vi "configure channel.vi"(7 "user event":T1, 8 "error in":errorcluster, 9 "line":T2, 10 "engine configuration in":refnum<class "engine configuration.lvclass">, 11 "Scan Engine configuration in":refnum<class "Scan Engine configuration.lvclass">) -> (0 "error out":errorcluster, 2 "engine configuration out":refnum<class "engine configuration.lvclass">, 3 "Scan Engine configuration out":refnum<class "Scan Engine configuration.lvclass">)   [LabVIEW 2013, in "Scan Engine editor node.lvclass"]
uses:
  Scan Engine editor node.lvclass
  module/configuration/Scan Engine configuration.lvclass
  <vilib>/NI/Module Execution Interface/Engine Configuration/engine configuration.lvclass
  table line.ctl
  <vilib>/NI/Tag Bus Module Framework/channel/TBM channel.lvclass
  <vilib>/NI/Configuration Framework/Node/UserEventRef.ctl
  <vilib>/NI/Configuration Framework/Controls/EventCluster.ctl
  <vilib>/NI/Configuration Framework/serializable configuration/NISE_CEF_serializable configuration.lvclass/NISE_CEF_serializable configuration.ctl
  <vilib>/NI/Tag Bus/tag/tag descriptor.lvclass/tag descriptor.ctl
  <vilib>/Utility/LVClass/Get LV Class Name.vi
  <vilib>/NI/Configuration Framework/error generator/NISE_error generator.vi
  <vilib>/NI/Tag Bus/tag/tag descriptor.lvclass
  <vilib>/NI/Configuration Framework/NISE_CEF_TreeControl.lvlib
  <vilib>/NI/Configuration Framework/serializable configuration/NISE_CEF_serializable configuration.lvclass
  <vilib>/NI/Configuration Framework/Node/NISE_CEF_Node.lvclass
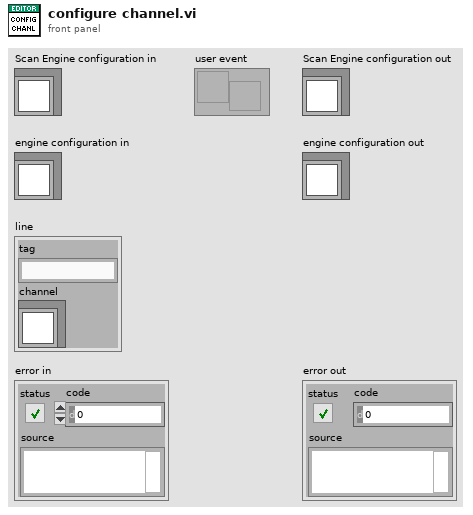
[diagram p1: front panel]
types:
  T1 = typedef "NISE_CEF_Node.lvclass/UserEventRef.ctl" = refnum<user-event>
  T2 = typedef "Scan Engine editor node.lvclass/table line.ctl" = cluster{"tag":string, "channel":refnum<class "TBM channel.lvclass">}
  T3 = typedef "NISE_CEF_TreeControl.lvlib/EventCluster.ctl" = cluster{"command":string, "data":string}
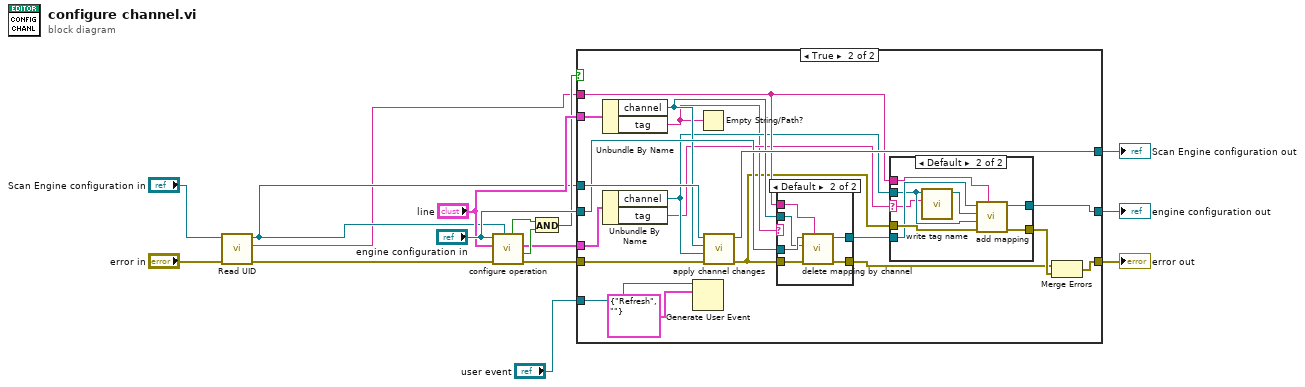
[diagram p0: block diagram]
diagram:
  n1 = call <vilib>:"Read UID.vi"("error in"="error in", "configuration in"="Scan Engine configuration in") -> ("error out"=w4:errorcluster, "instance id"=w1:string, "configuration out"=w2:refnum<class "Scan Engine configuration.lvclass">)  [unwired: 7 in]
  n2 = call "configure operation.vi"("Scan Engine configuration"=w2, "error in"=w4, "line item in"="line", "engine configuration in"="engine configuration in") -> ("error out"=w7:errorcluster, "success"=w12:bool, "line item out"=w8:T2, "changed"=w11:bool)  [unwired: 4 in]
  n3 = And(x=w11, y=w12) -> (x .and. y?=w13:bool)
  n4 = case shown="True" w13 {
    tunnel: [w18 w24] -> w10
    tunnel: [w19 w28] -> w15
    tunnel: "engine configuration in" -> [w19 w33]
    tunnel: w7 -> [w18 w35]
    tunnel: w8 -> [_ w38]
    tunnel: w2 -> [w17 w37]
    tunnel: [w17 w34] -> w9
    tunnel: w1 -> [_ w30]
    tunnel: "line" -> [_ w36]
    tunnel: "user event" -> [_ w20]
    frame False {
    }
    frame True {
      n5 = Unbundle By Name(w36) -> ("channel"=w32:refnum<class "TBM channel.lvclass">, "tag"=w25:string)
      n6 = Unbundle By Name(w38) -> ("channel"=w27:refnum<class "TBM channel.lvclass">, "tag"=w26:string)
      n7 = Generate User Event(user event=w20, event data cluster=T3 {"command"="Refresh", "data"=""} ("event data")) -> ()  [unwired: 2 in, 2 out]
      n8 = Empty String/Path?(string/path=w25) -> ()  [unwired: 1 out]
      n9 = call "apply channel changes.vi"("error in"=w35, "new"=w27, "old"=w32, "Scan Engine configuration"=w37) -> ("error out"=w22:errorcluster, "Scan Engine configuration out"=w34:refnum<class "Scan Engine configuration.lvclass">)  [unwired: 6 in]
      n10 = case shown="Default" w25 {
        tunnel: w22 -> [w39 w46]
        tunnel: w33 -> [w40 w45]
        tunnel: w32 -> [_ w44]
        tunnel: [w39 w43] -> w23
        tunnel: w30 -> [_ w42]
        tunnel: [w40 w41] -> w29
        frame "" {
        }
        frame Default {
          n11 = call <vilib>:"delete mapping by channel.vi"("owner ID"=w42, "error in"=w46, "channel"=w44, "engine configuration in"=w45) -> ("error out"=w43:errorcluster, "engine configuration out"=w41:refnum<class "engine configuration.lvclass">)  [unwired: 6 in]
        }
      }
      n12 = case shown="Default" w26 {
        selector: w26 -> [_ w49]
        tunnel: w22 -> [w47 w56]
        tunnel: [w47 w55] -> w31
        tunnel: w30 -> [_ w54]
        tunnel: w29 -> [w48 w53]
        tunnel: [w48 w52] -> w28
        tunnel: w27 -> [_ w50]
        frame "" {
        }
        frame Default {
          n13 = call <vilib>:"write tag name.vi"("name"=w49, "system tag in"=w50) -> ("system tag out"=w51:refnum<class "TBM channel.lvclass">)  [unwired: 8 in, 1 out]
          n14 = call <vilib>:"add mapping.vi"("owner ID"=w54, "error in"=w56, "channel"=w50, "tag descriptor"=w51, "engine configuration"=w53) -> ("error out"=w55:errorcluster, "engine configuration out"=w52:refnum<class "engine configuration.lvclass">)  [unwired: 5 in]
        }
      }
      n15 = Merge Errors(w23, w31) -> (w24:errorcluster)
    }
  }
  "engine configuration out" <- w15
  "error out" <- w10
  "Scan Engine configuration out" <- w9
